vi "Get Config Properties.vi"(8 "error in (no error)":errorcluster, 11 "RunningAverageCalculation in":refnum<class "RunningAverageCalculation.lvclass">) -> (0 "error out":errorcluster, 3 "RunningAverageCalculation out":refnum<class "RunningAverageCalculation.lvclass">)   [LabVIEW 2015, in "RunningAverageCalculation.lvclass"]
uses:
  Waveform-Processing-Custom-Device Configuration.llb/RunningAverageCalculation.lvclass
  Waveform-Processing-Custom-Device Configuration.llb/WaveformCalculation.lvclass
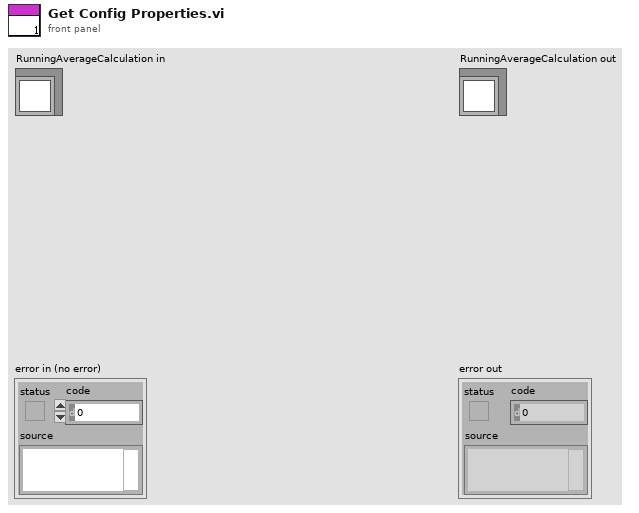
[diagram p1: front panel]
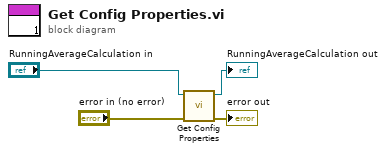
[diagram p0: block diagram]
diagram:
  n1 = call-parent "Get Config Properties.vi"("error in (no error)"="error in (no error)", "WaveformCalculation in"="RunningAverageCalculation in") -> ("error out"=→"error out":errorcluster, "WaveformCalculation out"=→"RunningAverageCalculation out":refnum<class "RunningAverageCalculation.lvclass">)  [unwired: 8 in]
